vi "Allocate Block.vi"   [LabVIEW 2016, in "GE 5565PIORC.lvclass"]
uses:
  GE 5565PIORC.lvclass
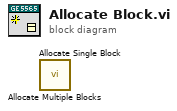
[diagram p0: block diagram]
diagram:
  n1 = call "Allocate Multiple Blocks.vi"() -> ()  [unwired: 9 in, 3 out]
  n2 = call "Allocate Single Block.vi"() -> ()  [unwired: 9 in, 3 out]
